vi "FileInfo_Global.vi"() -> ()   [LabVIEW 2015]
panel:
  in  "File Index":u32 format="%04d"
  in  "Lock File Number":bool
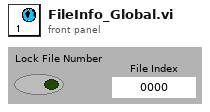
[diagram p1: front panel]
diagram:
